vi "LDO Line Transient - Flat.vi"(11 "error in (no error)":errorcluster) -> (15 "error out":errorcluster)   [LabVIEW 2020]
uses:
  <instrlib>/niScope/Controls/niScope vertical coupling.ctl
  <instrlib>/niScope/Controls/niScope trigger source digital.ctl
  <instrlib>/niDCPower/nidcpower.llb/niDCPower Aperture Time Units.ctl
  <instrlib>/niDCPower/nidcpower.llb/niDCPower Source Mode.ctl
  <instrlib>/niDCPower/nidcpower.llb/niDCPower Output Function.ctl
  <instrlib>/niDCPower/nidcpower.llb/niDCPower Export Signal - Signal.ctl
  <instrlib>/niDCPower/nidcpower.llb/niDCPower Wait For Event - Event.ctl
  <instrlib>/niScope/Controls/niScope trigger slope.ctl
  <instrlib>/niScope/Configure/Trigger/niScope Configure Trigger Digital.vi
  <instrlib>/niScope/Acquire/Fetch/niScope Multi Fetch Cluster.vi
  <instrlib>/niScope/Utility/niScope Get Channel Name From String.vi
  <vilib>/gmath/NI_Gmath.lvlib
  LDO Line Transient.lvlib
  <vilib>/gmath/NumericalOptimization/Nonlinear Curve Fit LM formula string.vi
panel:
  out "Horizontal:Number of Records":i32=400000
  out "Horizontal:Min Sample Rate":dbl=1000000.0
  out "Measurement:Measure Record Length":i32=10
  out "Measurement:Aperture Time":dbl=4.9999999999999996e-06
  out "Source:Advanced:Source Delay":dbl=3.086419753086419e-08
  in  "Tab Control":T1(tab)=enum."Waveform"
  in  "Scope":refnum<k15>="PXI1Slot5"
  in  "Load SMU":refnum<k15>="SMU1"
  in  "Source SMU":refnum<k15>="SMU1"
  in  "Load SMU Voltage Limit (V)":dbl=8.0
  in  "Load SMU Voltage Limit Range (V)":dbl=8.0
  in  "Load SMU Current Level Range (A)":dbl=3.0
  in  "Load SMU Channel":string="1"
  in  "Load Current (A)":dbl=-0.05
  in  "Min. Record Length":i32=400000
  in  "Min. Sampling Rate":dbl=1000000.0
  in  "Trigger Modifier":i32(ring) items=["None", "Auto"]
  in  "Reference Position":dbl
  in  "Input Impedance":u32(ring) items=["1 Mega Ohm"=0, "50 Ohm"=2]
  in  "Trigger Delay (sec)":dbl
  in  "Max. Input Frequency (Hz)":dbl
  in  "Vertical Offset (V)":dbl
  in  "Probe Attentuation":dbl=1.0
  in  "Vertical Range (V)":dbl=5.0
  in  "Scope Channel":string="0"
  in  "Source SMU Current Limit (A)":dbl=0.2
  in  "Source SMU Transient Response":i32(ring)=1039 items=["Slow"=1041, "Normal"=1038, "Fast"=1039, "Custom"=1042]
  in  "Source SMU Record Length":i32=10
  in  "Source SMU Aperture Time (sec)":dbl=5e-06
  in  "Source SMU Current Limit Range (A)":dbl=0.2
  in  "Source SMU Voltage Level Range (V)":dbl=8.0
  in  "Source SMU Channel":string="0"
  in  "Source  SMU Steady State Voltage (V)":dbl=4.0
  in  "Vertical Coupling":T2 items=["AC", "DC", "Ground"]
  in  "Trigger Source":T3="VAL_PFI_0" caption="trigger source (RTSI 0)"
  in  "Recovery Level (V)":dbl=0.1
  in  "Vin2 Voltage Level Width (sec)":dbl=0.1
  in  "Source Voltage 2 - Vin2":dbl=5.0
  in  "Source Voltage 1 - Vin1":dbl=4.0
  out "Settling time (ms)":dbl=0.008841
  out "Mixed Signal Graph":cluster{waveform(dbl), waveform(dbl)}(graph)={{"t0"=timestamp(0 s since 1904-01-01), "dt"=4.9999999999999996e-06, "Y"=array[40000 elements]}, {"t0"=timestamp(0 s since 1904-01-01), "dt"=4.9999999999999996e-06, "Y"=array[40000 elements]}}
  out "Waveform Graph":dbl[](graph)
  out "Waveform(s)":T4(graph)={"relativeInitialX"=1e-06, "xIncrement"=1e-06, "wfm"=array[400000 elements]} caption="Instantaneous Load Transient Waveform"
  out "XY Graph 2":cluster{dbl[], dbl[]}[](graph)
  out "XY Graph":cluster{dbl[], "wfm":dbl[]}[](graph)
  # "Line Transient Measurement - Flat VI"
  # "Source SMU Config"
  # "Scope Config"
  # "Load SMU Config"
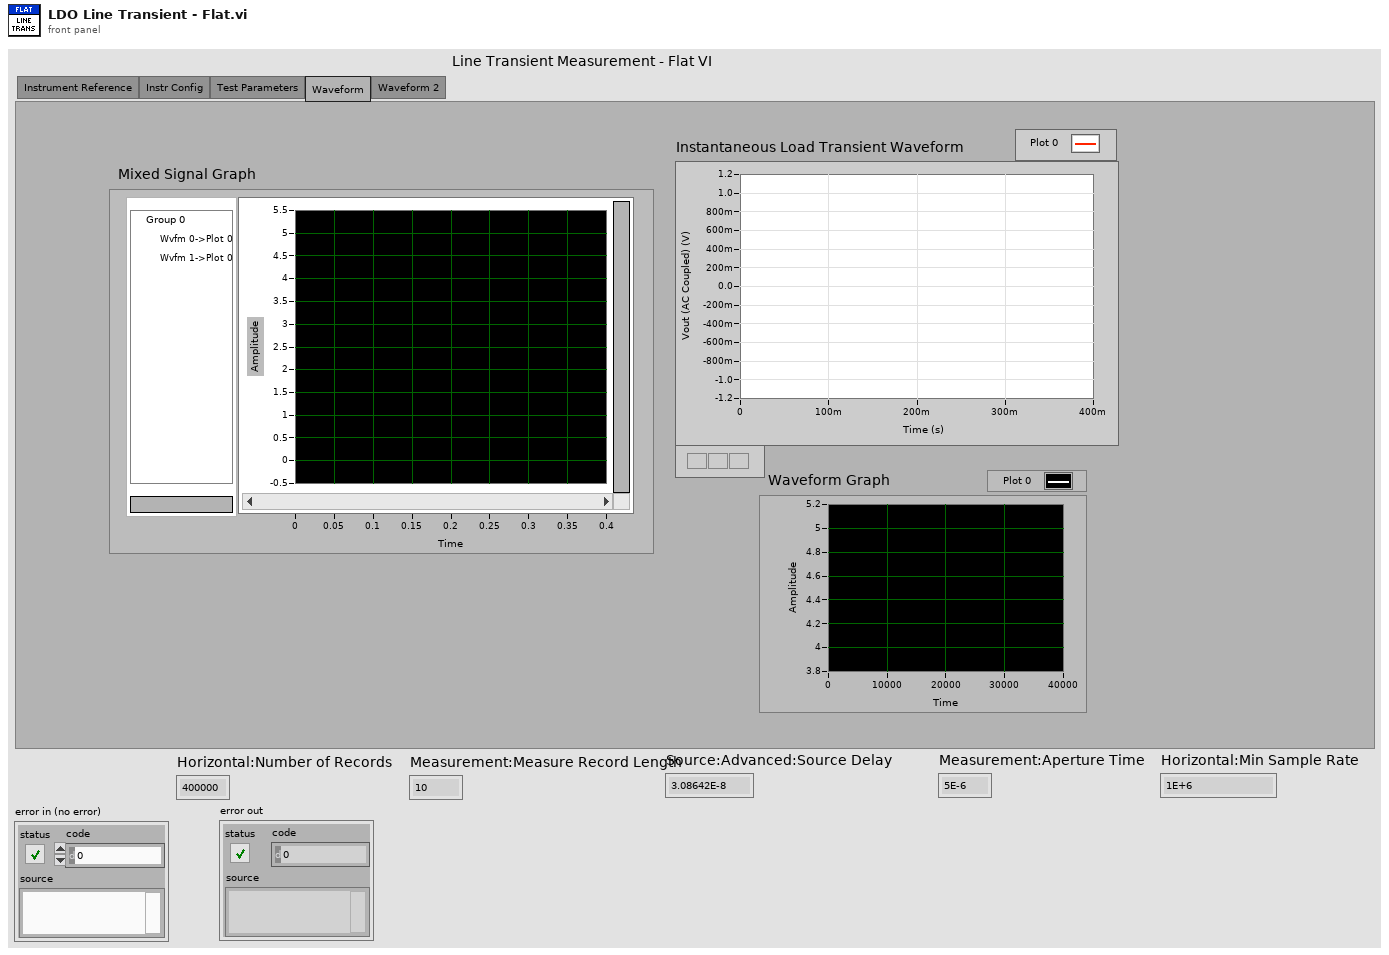
[diagram p1: front panel]
types:
  T1 = enum32{"Instrument Reference", "Instr Config", "Test Parameters", "Waveform", "Waveform 2"}
  T2 = typedef "niScope vertical coupling.ctl" = i32
  T3 = typedef "niScope trigger source digital.ctl" = string
  T4 = cluster{"relativeInitialX":dbl, "xIncrement":dbl, "wfm":dbl[]}
  T5 = typedef "niDCPower Output Function.ctl" = i32
  T6 = typedef "niDCPower Source Mode.ctl" = i32
  T7 = typedef "niScope trigger slope.ctl" = i32
  T8 = typedef "niDCPower Wait For Event - Event.ctl" = i32
  T9 = typedef "niDCPower Export Signal - Signal.ctl" = i32
  T10 = typedef "niDCPower Aperture Time Units.ctl" = i32
  T11 = cluster{"relativeInitialX":dbl, "xIncrement":dbl, "wfm":dbl[]}[]
  T12 = cluster{"model":string, "Parameters":string[], "x":string}
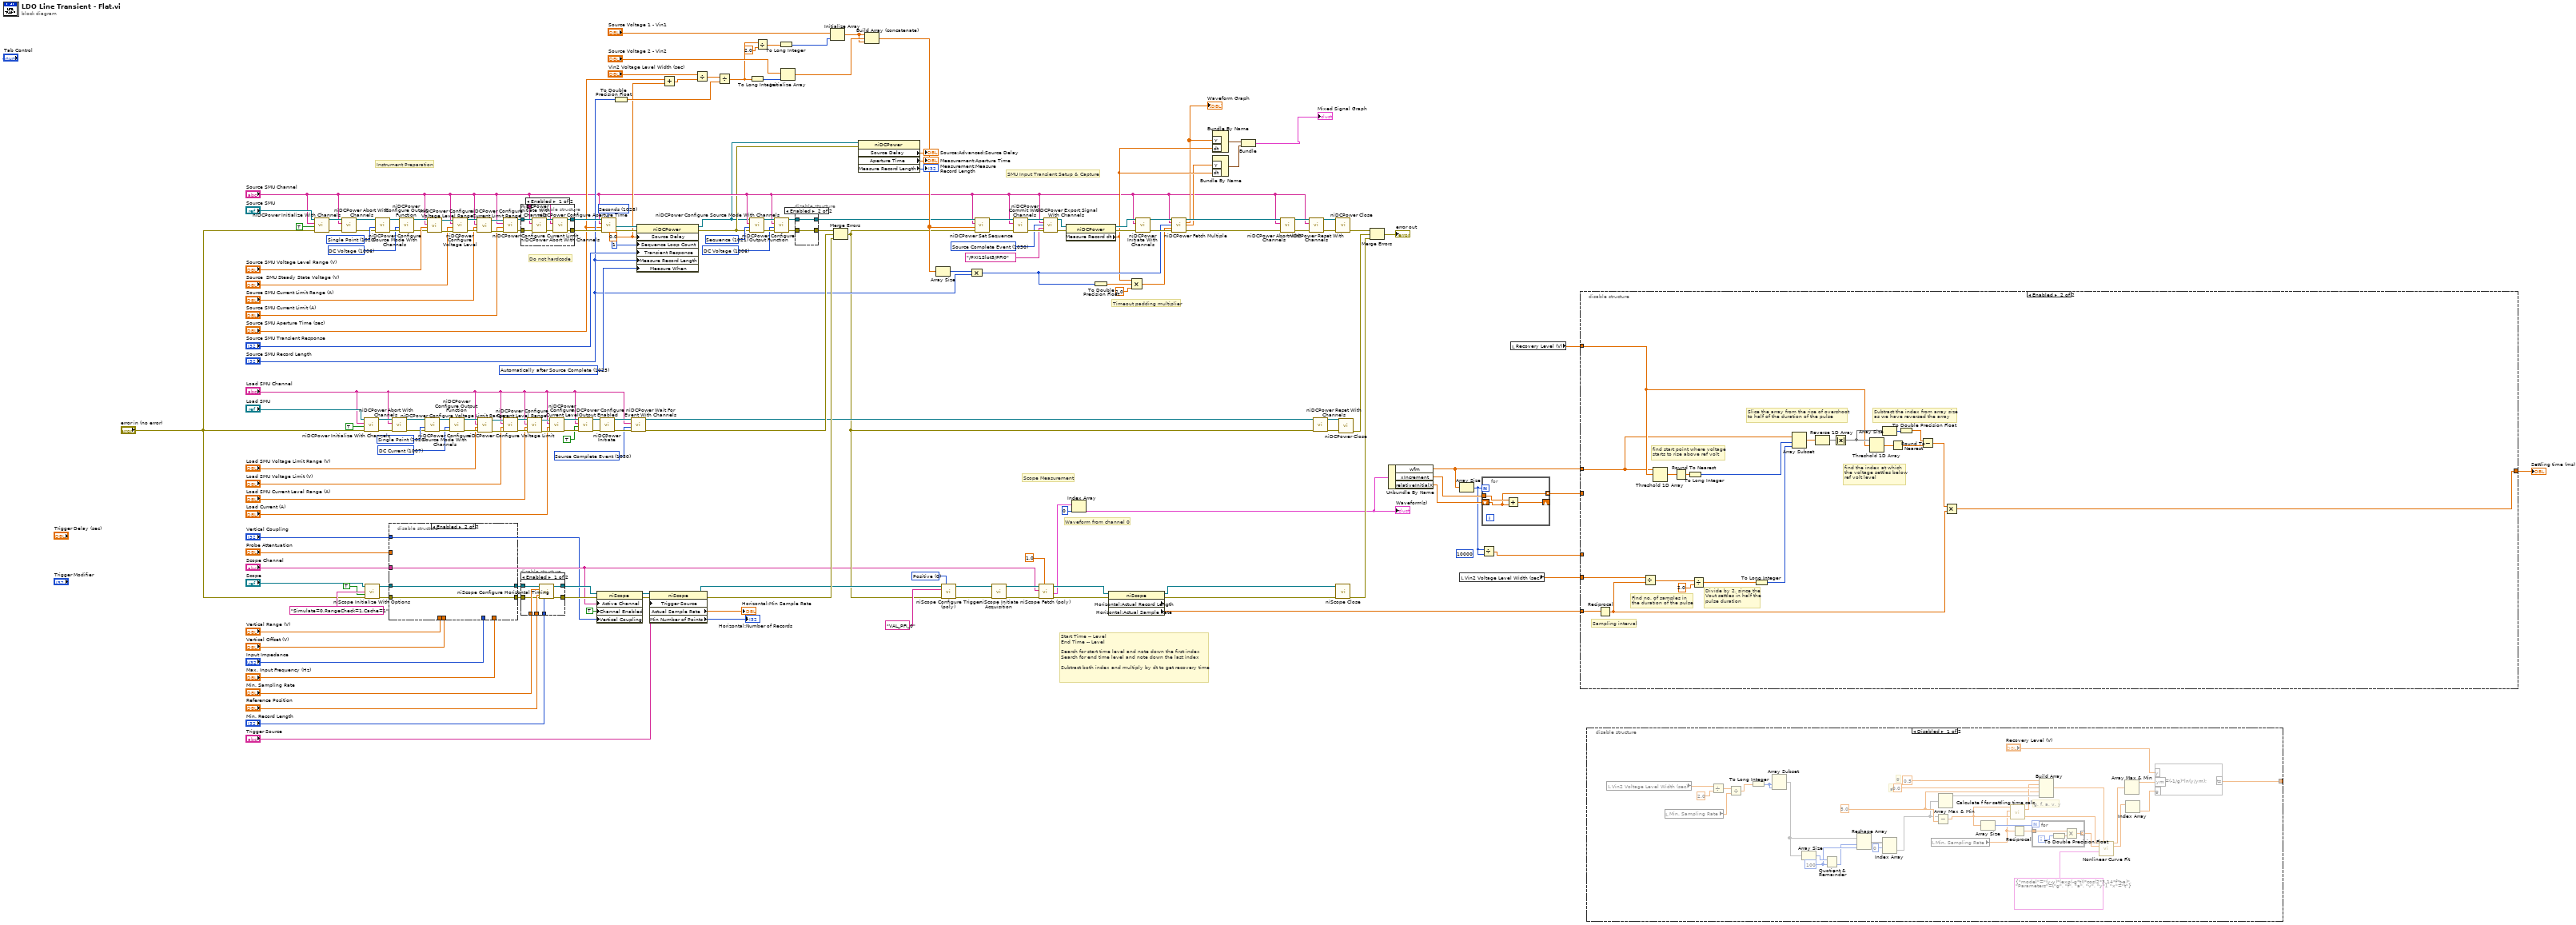
[diagram p0: block diagram]
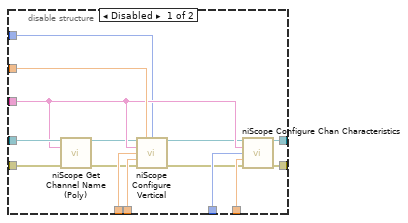
[diagram p2: hidden frame]
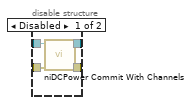
[diagram p4: hidden frame]
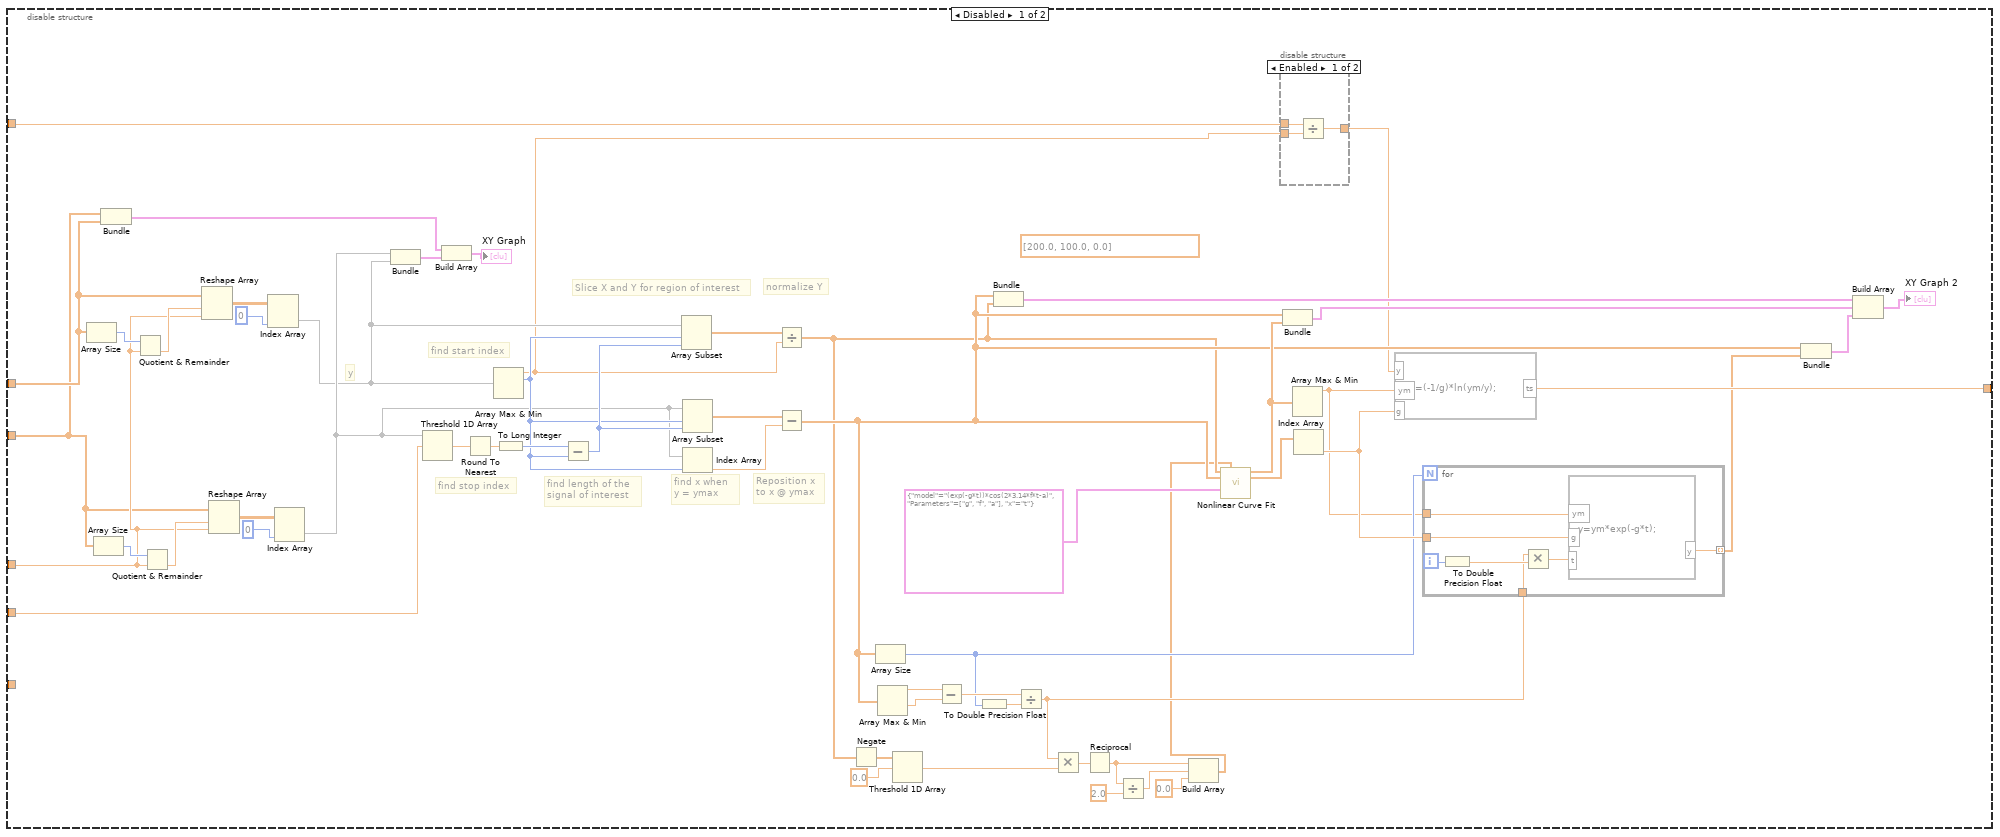
[diagram p5: hidden frame]
diagram:
  (unwired) 10000 ("y")
  w49 = T5 1006 items=["DC Voltage"=1006, "DC Current"=1007, "Pulse Voltage"=1049, "Pulse Current"=1050] ("output function")
  w50 = T6 1021 items=["Single Point"=1020, "Sequence"=1021] ("source mode")
  w43 = T7 0 items=["Positive", "Negative"] ("trigger slope")
  w76 = T8 1030 items=["Source Complete Event"=1030, "Measure Complete Event"=1031, "Sequence Iteration Complete Event"=1032, "Sequence Engine Done Event"=1033, "Pulse Complete Event"=1051, "Ready For Pulse Trigger Event"=1052] ("event")
  w110 = T9 1030 items=["Source Complete Event"=1030, "Measure Complete Event"=1031, "Sequence Iteration Complete Event"=1032, "Sequence Engine Done Event"=1033, "Pulse Complete Event"=1051, "Ready For Pulse Trigger Event"=1052, "Start Trigger"=1034, "Source Trigger"=1035, "Measure Trigger"=1036, "Sequence Advance Trigger"=1037, "Pulse Trigger"=1053] ("signal")
  w150 = T5 1007 items=["DC Voltage"=1006, "DC Current"=1007, "Pulse Voltage"=1049, "Pulse Current"=1050] ("output function")
  w151 = T6 1020 items=["Single Point"=1020, "Sequence"=1021] ("source mode")
  w159 = 1025 items=["Automatically after Source Complete"=1025, "On Demand"=1026, "On Measure Trigger"=1027] ("Measurement:Advanced:Measure When")
  w34 = 0.0 ("Source:Advanced:Source Delay")
  w166 = T10 1028 items=["Seconds"=1028, "Powerline Cycles"=1029] ("aperture time units")
  w169 = T5 1006 items=["DC Voltage"=1006, "DC Current"=1007, "Pulse Voltage"=1049, "Pulse Current"=1050] ("output function")
  w170 = T6 1020 items=["Single Point"=1020, "Sequence"=1021] ("source mode")
  # "Do not hardcode"
  # "Start Time -- Level\nEnd Time -- Level\n\nSearch for start time level and note down the first index\nSearch for end time level and note down the last index\n\nSubtract both index and multiply by dt to get recovery time"
  # "SMU Input Transient Setup & Capture"
  # "Scope Measurement"
  # "Waveform from channel 0"
  # "Timeout padding multiplier"
  # "Instrument Preparation"
  n1 = call <instrlib>:"niDCPower Initialize With Channels.vi"("error in (no error)"="error in (no error)", "reset (false)"=TRUE, "channels"="Source SMU Channel", "resource name"="Source SMU") -> ("error out"=w165:errorcluster, "instrument handle out"=w163:refnum<k15>)  [unwired: 1 in, 5 out]
  n2 = call <instrlib>:"niDCPower Abort With Channels.vi"("error in (no error)"=w165, "channel name"="Source SMU Channel", "instrument handle"=w163) -> ("error out"=w164:errorcluster, "instrument handle out"=w162:refnum<k15>)  [unwired: 7 in]
  n3 = call <instrlib>:"niDCPower Initialize With Channels.vi"("error in (no error)"="error in (no error)", "reset (false)"=TRUE, "channels"="Load SMU Channel", "resource name"="Load SMU") -> ("error out"=w147:errorcluster, "instrument handle out"=w145:refnum<k15>)  [unwired: 1 in, 5 out]
  n4 = call <instrlib>:"niScope Initialize With Options.vi"("resource name"="Scope", "option string"="Simulate=0,RangeCheck=1,Cache=1", "reset device"=TRUE, "error in"="error in (no error)") -> ("instrument handle"=w136:refnum<k15>, "error out"=w135:errorcluster)  [unwired: 10 in]
  n5 = call <instrlib>:"niDCPower Configure Source Mode With Channels.vi"("error in (no error)"=w164, "source mode"=w170, "instrument handle"=w162) -> ("error out"=w171:errorcluster, "instrument handle out"=w172:refnum<k15>)  [unwired: 7 in]
  n6 = disable-structure shown="Enabled" {
    disable-tunnel: w136 -> [w199 w200]
    disable-tunnel: w135 -> [w198 w201]
    disable-tunnel: "Probe Attentuation" -> [w197 _]
    disable-tunnel: "Vertical Range (V)" -> [w196 _]
    disable-tunnel: "Vertical Offset (V)" -> [w195 _]
    disable-tunnel: "Max. Input Frequency (Hz)" -> [w194 _]
    disable-tunnel: "Input Impedance" -> [w193 _]
    disable-tunnel: "Scope Channel" -> [w192 _]
    disable-tunnel: "Vertical Coupling" -> [w191 _]
    disable-tunnel: [w186 w201] -> w2
    disable-tunnel: [w185 w200] -> w1
    frame Disabled {
      n7 = call-poly <instrlib>:"niScope Get Channel Name (Poly).vi"("instrument handle"=w199, "index"=w192, "error in"=w198) -> ("instrument handle out"=w190:refnum<k15>, "error out"=w189:errorcluster)  [unwired: 10 in, 1 out]
      n8 = call <instrlib>:"niScope Configure Vertical.vi"("instrument handle"=w190, "probe attenuation"=w197, "vertical coupling"=w191, "channels"=w192, "vertical range"=w196, "vertical offset"=w195, "error in"=w189) -> ("instrument handle out"=w188:refnum<k15>, "error out"=w187:errorcluster)  [unwired: 7 in]
      n9 = call <instrlib>:"niScope Configure Chan Characteristics.vi"("instrument handle"=w188, "channels"=w192, "input impedance"=w193, "maximum input frequency"=w194, "error in"=w187) -> ("instrument handle out"=w185:refnum<k15>, "error out"=w186:errorcluster)  [unwired: 9 in]
    }
    frame Enabled {
    }
  }
  n10 = call <instrlib>:"niDCPower Abort With Channels.vi"("error in (no error)"=w147, "channel name"="Load SMU Channel", "instrument handle"=w145) -> ("error out"=w146:errorcluster, "instrument handle out"=w144:refnum<k15>)  [unwired: 7 in]
  n11 = call <instrlib>:"niDCPower Configure Output Function.vi"("error in (no error)"=w171, "output function"=w169, "instrument handle"=w172) -> ("error out"=w167:errorcluster, "instrument handle out"=w168:refnum<k15>)  [unwired: 7 in]
  n12 = call <instrlib>:"niDCPower Configure Source Mode With Channels.vi"("error in (no error)"=w146, "source mode"=w151, "instrument handle"=w144) -> ("error out"=w152:errorcluster, "instrument handle out"=w153:refnum<k15>)  [unwired: 7 in]
  n13 = call <instrlib>:"niDCPower Configure Voltage Level Range.vi"("error in (no error)"=w167, "voltage level range"="Source SMU Voltage Level Range (V)", "channel name"="Source SMU Channel", "instrument handle"=w168) -> ("error out"=w184:errorcluster, "instrument handle out"=w183:refnum<k15>)  [unwired: 6 in]
  n14 = call <instrlib>:"niDCPower Configure Output Function.vi"("error in (no error)"=w152, "output function"=w150, "instrument handle"=w153) -> ("error out"=w148:errorcluster, "instrument handle out"=w149:refnum<k15>)  [unwired: 7 in]
  n15 = call <instrlib>:"niDCPower Configure Voltage Level.vi"("error in (no error)"=w184, "voltage level"="Source  SMU Steady State Voltage (V)", "channel name"="Source SMU Channel", "instrument handle"=w183) -> ("error out"=w182:errorcluster, "instrument handle out"=w181:refnum<k15>)  [unwired: 6 in]
  n16 = call <instrlib>:"niDCPower Configure Current Limit Range.vi"("error in (no error)"=w182, "current limit range"="Source SMU Current Limit Range (A)", "channel name"="Source SMU Channel", "instrument handle"=w181) -> ("error out"=w180:errorcluster, "instrument handle out"=w179:refnum<k15>)  [unwired: 6 in]
  n17 = call <instrlib>:"niDCPower Configure Voltage Limit Range.vi"("error in (no error)"=w148, "voltage limit range"="Load SMU Voltage Limit Range (V)", "channel name"="Load SMU Channel", "instrument handle"=w149) -> ("error out"=w158:errorcluster, "instrument handle out"=w157:refnum<k15>)  [unwired: 6 in]
  n18 = call <instrlib>:"niDCPower Configure Current Limit.vi"("error in (no error)"=w180, "current limit"="Source SMU Current Limit (A)", "channel name"="Source SMU Channel", "instrument handle"=w179) -> ("error out"=w47:errorcluster, "instrument handle out"=w45:refnum<k15>)  [unwired: 6 in]
  n19 = call <instrlib>:"niDCPower Configure Voltage Limit.vi"("error in (no error)"=w158, "voltage limit"="Load SMU Voltage Limit (V)", "channel name"="Load SMU Channel", "instrument handle"=w157) -> ("error out"=w156:errorcluster, "instrument handle out"=w155:refnum<k15>)  [unwired: 6 in]
  n20 = disable-structure shown="Enabled" {
    disable-tunnel: w47 -> [w206 w209]
    disable-tunnel: [w205 w209] -> w46
    disable-tunnel: w45 -> [w204 w210]
    disable-tunnel: [w203 w210] -> w44
    disable-tunnel: "Source SMU Channel" -> [w202 _]
    frame Enabled {
      n21 = call <instrlib>:"niDCPower Initiate With Channels.vi"("error in (no error)"=w206, "channel name"=w202, "instrument handle"=w204) -> ("error out"=w208:errorcluster, "instrument handle out"=w207:refnum<k15>)  [unwired: 7 in]
      n22 = call <instrlib>:"niDCPower Abort With Channels.vi"("error in (no error)"=w208, "channel name"=w202, "instrument handle"=w207) -> ("error out"=w205:errorcluster, "instrument handle out"=w203:refnum<k15>)  [unwired: 7 in]
    }
    frame Disabled {
    }
  }
  n23 = disable-structure shown="Enabled" {
    disable-tunnel: "Min. Record Length" -> [w217 _]
    disable-tunnel: "Reference Position" -> [w216 _]
    disable-tunnel: "Min. Sampling Rate" -> [w215 _]
    disable-tunnel: [w214 w218] -> w11
    disable-tunnel: [w213 w219] -> w9
    disable-tunnel: w2 -> [w212 w218]
    disable-tunnel: w1 -> [w211 w219]
    frame Enabled {
      n24 = call <instrlib>:"niScope Configure Horizontal Timing.vi"("instrument handle"=w211, "min sample rate"=w215, "reference position"=w216, "error in"=w212, "min record length"=w217) -> ("instrument handle out"=w213:refnum<k15>, "error out"=w214:errorcluster)  [unwired: 9 in]
    }
    frame Disabled {
    }
  }
  n25 = call <instrlib>:"niDCPower Configure Current Level Range.vi"("error in (no error)"=w156, "current level range"="Load SMU Current Level Range (A)", "channel name"="Load SMU Channel", "instrument handle"=w155) -> ("error out"=w141:errorcluster, "instrument handle out"=w142:refnum<k15>)  [unwired: 6 in]
  n26 = call <instrlib>:"niDCPower Configure Current Level.vi"("error in (no error)"=w141, "current level"="Load Current (A)", "channel name"="Load SMU Channel", "instrument handle"=w142) -> ("error out"=w81:errorcluster, "instrument handle out"=w78:refnum<k15>)  [unwired: 6 in]
  n27 = call <instrlib>:"niDCPower Configure Output Enabled.vi"("error in (no error)"=w81, "output enabled"=TRUE, "channel name"="Load SMU Channel", "instrument handle"=w78) -> ("error out"=w80:errorcluster, "instrument handle out"=w83:refnum<k15>)  [unwired: 6 in]
  n28 = property class="niScope"(reference=w9, error in=w11, "Active Channel"="Scope Channel", "Channel Enabled"=TRUE ("Vertical:Channel Enabled"), "Vertical Coupling"="Vertical Coupling") -> (reference out=w8:refnum<k15>, error out=w10:errorcluster)
  n29 = call <instrlib>:"niDCPower Initiate.vi"("error in (no error)"=w80, "instrument handle"=w83) -> ("error out"=w79:errorcluster, "instrument handle out"=w82:refnum<k15>)  [unwired: 8 in]
  n30 = call <instrlib>:"niDCPower Configure Aperture Time.vi"("aperture time units"=w166, "error in (no error)"=w46, "aperture time"="Source SMU Aperture Time (sec)", "channel name"="Source SMU Channel", "instrument handle"=w44) -> ("error out"=w84:errorcluster, "instrument handle out"=w41:refnum<k15>)  [unwired: 5 out]
  n31 = To Double Precision Float(number="Source SMU Record Length") -> (double precision float=w38:dbl)
  n32 = call <instrlib>:"niDCPower Wait For Event With Channels.vi"("error in (no error)"=w79, "event"=w76, "channel name"="Load SMU Channel", "instrument handle"=w82) -> ("error out"=w74:errorcluster, "instrument handle out"=w57:refnum<k15>)  [unwired: 6 in]
  n33 = property class="niDCPower"(reference=w41, error in=w84, "Source Delay"=w34, "Sequence Loop Count"=1 ("Source:Advanced:Sequence Loop Count"), "Transient Response"="Source SMU Transient Response", "Measure Record Length"="Source SMU Record Length", "Measure When"=w159) -> (reference out=w12:refnum<k15>, error out=w13:errorcluster)
  n34 = property class="niScope"(reference=w8, error in=w10, "Trigger Source"="Trigger Source") -> (reference out=w71:refnum<k15>, error out=w73:errorcluster, "Actual Sample Rate"=→"Horizontal:Min Sample Rate":dbl, "Min Number of Points"=→"Horizontal:Number of Records":i32)
  n35 = Add(x="Source SMU Aperture Time (sec)", y=w34) -> (x+y=w35:dbl)
  n36 = Divide(x="Vin2 Voltage Level Width (sec)", y=w35) -> (x/y=w40:dbl)
  n37 = Divide(x=w40, y=w38) -> (x/y=w37:dbl)
  n38 = call <instrlib>:"niDCPower Configure Source Mode With Channels.vi"("error in (no error)"=w13, "source mode"=w50, "channel name"="Source SMU Channel", "instrument handle"=w12) -> ("error out"=w51:errorcluster, "instrument handle out"=w48:refnum<k15>)  [unwired: 6 in]
  n39 = To Long Integer(number=w37) -> (32bit integer=w122:i32)
  n40 = Divide(x=w37, y=2.0) -> (x/y=w118:dbl)
  n41 = call <instrlib>:"niDCPower Configure Output Function.vi"("error in (no error)"=w51, "output function"=w49, "channel name"="Source SMU Channel", "instrument handle"=w48) -> ("error out"=w18:errorcluster, "instrument handle out"=w16:refnum<k15>)  [unwired: 6 in]
  n42 = To Long Integer(number=w118) -> (32bit integer=w117:i32)
  n43 = Initialize Array("Source Voltage 2 - Vin2", w122) -> (w116:dbl[])
  n44 = disable-structure shown="Enabled" {
    disable-tunnel: w18 -> [w223 w224]
    disable-tunnel: [w222 w224] -> w17
    disable-tunnel: w16 -> [w221 w225]
    disable-tunnel: [w220 w225] -> w15
    frame Disabled {
      n45 = call <instrlib>:"niDCPower Commit With Channels.vi"("error in (no error)"=w223, "instrument handle"=w221) -> ("error out"=w222:errorcluster, "instrument handle out"=w220:refnum<k15>)  [unwired: 8 in]
    }
    frame Enabled {
    }
  }
  n46 = Initialize Array("Source Voltage 1 - Vin1", w117) -> (w115:dbl[])
  n47 = Merge Errors(w17, w74, w73) -> (w22:errorcluster)
  n48 = property class="niDCPower"(reference=w12, error in=w13) -> ("Source Delay"=→"Source:Advanced:Source Delay":dbl, "Aperture Time"=→"Measurement:Aperture Time":dbl, "Measure Record Length"=→"Measurement:Measure Record Length":i32)  [unwired: 2 out]
  n49 = Build Array (concatenate)(w115, w116, w115) -> (w106:dbl[])
  n50 = Array Size(array=w106) -> (size(s)=w105:i32)
  n51 = call-poly <instrlib>:"niScope Configure Trigger (poly).vi"("instrument handle"=w71, "trigger slope"=w43, "trigger source"=T3 "VAL_PFI_0", "error in"=w22) -> ("instrument handle out"=w72:refnum<k15>, "error out"=w86:errorcluster)  [unwired: 10 in]
  n52 = Compound Arithmetic op=MULTIPLY(w105, "Source SMU Record Length") -> (w98:i32)
  n53 = call <instrlib>:"niDCPower Set Sequence.vi"("error in (no error)"=w22, "values"=w106, "channel name"="Source SMU Channel", "instrument handle"=w15) -> ("error out"=w114:errorcluster, "instrument handle out"=w113:refnum<k15>)  [unwired: 1 in, 5 out]
  n54 = call <instrlib>:"niScope Initiate Acquisition.vi"("instrument handle"=w72, "error in"=w86) -> ("instrument handle out"=w69:refnum<k15>, "error out"=w85:errorcluster)  [unwired: 12 in]
  n55 = call <instrlib>:"niDCPower Commit With Channels.vi"("error in (no error)"=w114, "channel name"="Source SMU Channel", "instrument handle"=w113) -> ("error out"=w112:errorcluster, "instrument handle out"=w111:refnum<k15>)  [unwired: 7 in]
  n56 = call-poly <instrlib>:"niScope Fetch (poly).vi"("timeout"=1.0, "error in"=w85, "channels"="Scope Channel", "instrument handle"=w69) -> ("error out"=w87:errorcluster, "waveform"=w66:T11, "instrument handle out"=w67:refnum<k15>)  [unwired: 4 in, 1 out]
  n57 = call <instrlib>:"niDCPower Export Signal With Channels.vi"("instrument handle"=w111, "channel name"="Source SMU Channel", "signal"=w110, "output terminal"=tag "/PXI1Slot5/PFI0", "error in (no error)"=w112) -> ("instrument handle out"=w107:refnum<k15>, "error out"=w108:errorcluster)  [unwired: 9 in]
  n58 = property class="niDCPower"(reference=w107, error in=w108) -> (reference out=w101:refnum<k15>, error out=w102:errorcluster, "Measure Record dt"=w90:dbl)
  n59 = Index Array(array=w66, index=0) -> (element=w33:T4)
  "Waveform(s)" <- w33
  n60 = To Double Precision Float(number=w98) -> (double precision float=w103:dbl)
  n61 = property class="niScope" props=["Horizontal:Actual Record Length", "Horizontal:Actual Sample Rate"](reference=w67, error in=w87) -> (reference out=w63:refnum<k15>, error out=w64:errorcluster, "Horizontal:Actual Sample Rate"=w23:dbl)  [unwired: 1 out]
  n62 = Compound Arithmetic op=MULTIPLY(w90, w103, 2.0 ("value")) -> (w97:dbl)
  n63 = call <instrlib>:"niDCPower Initiate With Channels.vi"("error in (no error)"=w102, "channel name"="Source SMU Channel", "instrument handle"=w101) -> ("error out"=w100:errorcluster, "instrument handle out"=w99:refnum<k15>)  [unwired: 7 in]
  n64 = call <instrlib>:"niDCPower Fetch Multiple.vi"("instrument handle"=w99, "channel name"="Source SMU Channel", "count (1)"=w98, "timeout (sec)"=w97, "error in (no error)"=w100) -> ("instrument handle out"=w95:refnum<k15>, "voltage measurements"=w54:dbl[], "current measurements"=w89:dbl[], "error out"=w96:errorcluster)  [unwired: 7 out]
  "Waveform Graph" <- w54
  n65 = Bundle By Name("Y"=w54, "dt"=w90) -> (w88:waveform(dbl))  [unwired: 1 out]
  n66 = Bundle By Name("Y"=w89, "dt"=w90) -> (w53:waveform(dbl))  [unwired: 1 out]
  n67 = Bundle(w88, w53) -> (→"Mixed Signal Graph":cluster{waveform(dbl), waveform(dbl)})  [unwired: 1 in]
  n68 = call <instrlib>:"niDCPower Abort With Channels.vi"("error in (no error)"=w96, "channel name"="Source SMU Channel", "instrument handle"=w95) -> ("error out"=w93:errorcluster, "instrument handle out"=w91:refnum<k15>)  [unwired: 7 in]
  n69 = call <instrlib>:"niDCPower Reset With Channels.vi"("error in (no error)"=w93, "channel name"="Source SMU Channel", "instrument handle"=w91) -> ("error out"=w92:errorcluster, "instrument handle out"=w94:refnum<k15>)  [unwired: 7 in]
  n70 = call <instrlib>:"niDCPower Reset With Channels.vi"("error in (no error)"=w22, "instrument handle"=w57) -> ("error out"=w58:errorcluster, "instrument handle out"=w59:refnum<k15>)  [unwired: 8 in]
  n71 = call <instrlib>:"niDCPower Close.vi"("error in (no error)"=w92, "instrument handle"=w94) -> ("error out"=w62:errorcluster)  [unwired: 9 out]
  n72 = call <instrlib>:"niScope Close.vi"("instrument handle"=w63, "error in"=w64) -> ("error out"=w61:errorcluster)  [unwired: 13 in]
  n73 = call <instrlib>:"niDCPower Close.vi"("error in (no error)"=w58, "instrument handle"=w59) -> ("error out"=w56:errorcluster)  [unwired: 9 out]
  n74 = Merge Errors(w62, w56, w61) -> (→"error out":errorcluster)
  n75 = Unbundle By Name(w33) -> ("wfm"=w28:dbl[], "xIncrement"=w31:dbl, "relativeInitialX"=w32:dbl)
  n76 = Array Size(array=w28) -> (size(s)=w26:i32)
  n77 = local read "Vin2 Voltage Level Width (sec)"() -> (w25:dbl)
  n78 = Divide(x=w26, y=w26) -> (x/y=w29:dbl)
  n79 = for {
    N: w26 -> [_]
    tunnel: w31 -> [w228]
    shift-right: [w227] -> _
    shift-left: w32 -> [w226]
    tunnel: [w226] -> w27 mode=indexing
    n80 = Add(x=w228, y=w226) -> (x+y=w227:dbl)
  }
  n81 = local read "Recovery Level (V)"() -> (w24:dbl)
  n82 = disable-structure shown="Enabled" {
    disable-tunnel: [w274 w300] -> w30
    disable-tunnel: w29 -> [w255 _]
    disable-tunnel: w28 -> [w238 w297]
    disable-tunnel: w27 -> [w237 _]
    disable-tunnel: w25 -> [w230 w296]
    disable-tunnel: w24 -> [w229 w298]
    disable-tunnel: w23 -> [_ w299]
    frame Disabled {
      (unwired) dbl[] [200.0, 100.0, 0.0] ("initial parameters")
      # "find x when \ny = ymax"
      # "Reposition x \nto x @ ymax"
      # "normalize Y"
      # "Slice X and Y for region of interest"
      # "find length of the \nsignal of interest"
      # "find stop index"
      # "find start index"
      # "y"
      n83 = Array Size(array=w238) -> (size(s)=w264:i32)
      n84 = Array Size(array=w237) -> (size(s)=w268:i32)
      n85 = Bundle(w237, "wfm"=w238) -> (w235:cluster{dbl[], "wfm":dbl[]})  [unwired: 1 in]
      n86 = Quotient & Remainder(x=w264, y=w255) -> (floor(x/y)=w263:dbl)  [unwired: 1 out]
      n87 = Quotient & Remainder(x=w268, y=w255) -> (floor(x/y)=w267:dbl)  [unwired: 1 out]
      n88 = Reshape Array(w238, w263, w255) -> (w262:dbl[][])
      n89 = Reshape Array(w237, w267, w255) -> (w266:dbl[][])
      n90 = Index Array(array=w262, index (col)=0 ("index (row)")) -> (element=w261:dbl[])  [unwired: 1 in]
      n91 = Index Array(array=w266, index (col)=0 ("index (row)")) -> (element=w265:dbl[])  [unwired: 1 in]
      n92 = Bundle(w265, "wfm"=w261) -> (w272:cluster{dbl[], "wfm":dbl[]})  [unwired: 1 in]
      n93 = Threshold 1D Array(2:w230, 3:w265) -> (0:w283:dbl)  [unwired: 1 in]
      n94 = Build Array(w235, w272) -> (→"XY Graph":cluster{dbl[], "wfm":dbl[]}[])
      n95 = Round To Nearest(number=w283) -> (nearest integer value=w284:dbl)
      n96 = Array Max & Min(array=w261) -> (max value=w233:dbl, max index (indices)=w278:i32)  [unwired: 2 out]
      n97 = To Long Integer(number=w284) -> (32bit integer=w282:i32)
      n98 = Subtract(x=w282, y=w278) -> (x-y=w281:i32)
      n99 = Array Subset(array=w261, index=w278, length=w281) -> (w280:dbl[])
      n100 = Array Subset(array=w265, index=w278, length=w281) -> (w279:dbl[])
      n101 = Index Array(array=w265, index=w278) -> (element=w277:dbl)
      n102 = Divide(x=w280, y=w233) -> (x/y=w248:dbl[])
      n103 = Subtract(x=w279, y=w277) -> (x-y=w254:dbl[])
      n104 = Negate(x=w248) -> (-x=w247:dbl[])
      n105 = Array Size(array=w254) -> (size(s)=w250:i32)
      n106 = Array Max & Min(array=w254) -> (max value=w253:dbl, min value=w252:dbl)  [unwired: 2 out]
      n107 = Threshold 1D Array(2:0.0 ("threshold y"), 3:w247) -> (0:w245:dbl)  [unwired: 1 in]
      n108 = Subtract(x=w253, y=w252) -> (x-y=w251:dbl)
      n109 = To Double Precision Float(number=w250) -> (double precision float=w249:dbl)
      n110 = Bundle(w254, w248) -> (w273:cluster{dbl[], dbl[]})  [unwired: 1 in]
      n111 = Divide(x=w251, y=w249) -> (x/y=w244:dbl)
      n112 = Multiply(x=w244, y=w245) -> (x*y=w243:dbl)
      n113 = Reciprocal(x=w243) -> (1/x=w242:dbl)
      n114 = Divide(x=w242, y=2.0) -> (x/y=w240:dbl)
      n115 = Build Array(w242, w240, 0.0 ("element")) -> (w231:dbl[])
      n116 = call-poly <vilib>:"Nonlinear Curve Fit.vi"("Y"=w248, "initial parameters"=w231, "X"=w254, "model description"=T12 {"model"="(exp(-g*t))*cos(2*3.14*f*t-a)", "Parameters"=["g", "f", "a"], "x"="t"}) -> ("best nonlinear fit"=w271:dbl[], "best fit parameters"=w275:dbl[])  [unwired: 7 in, 3 out]
      n117 = disable-structure shown="Enabled" {
        disable-tunnel: w229 -> [w287 w288]
        disable-tunnel: [w286 w288] -> w234
        disable-tunnel: w233 -> [w285 _]
        frame Enabled {
          n118 = Divide(x=w287, y=w285) -> (x/y=w286:dbl)
        }
        frame Disabled {
        }
      }
      n119 = Bundle(w254, "best nonlinear fit"=w271) -> (w269:cluster{dbl[], "best nonlinear fit":dbl[]})  [unwired: 1 in]
      n120 = Array Max & Min(array=w271) -> (max value=w232:dbl)  [unwired: 3 out]
      n121 = Index Array(array=w275) -> (element=w258:dbl)  [unwired: 1 in]
      n122 = formula code="ts =(-1/g)*ln(ym/y);"("y"=w234, "ym"=w232, "g"=w258) -> ("ts"=w274:dbl)
      n123 = for {
        N: w250 -> [_]
        tunnel: [w294] -> w257 mode=indexing
        tunnel: w258 -> [w291]
        tunnel: w232 -> [w290]
        tunnel: w244 -> [w289]
        i -> [w295]
        n124 = To Double Precision Float(number=w295) -> (double precision float=w292:dbl)
        n125 = Multiply(x=w289, y=w292) -> (x*y=w293:dbl)
        n126 = formula code="y=ym*exp(-g*t);"("g"=w291, "ym"=w290, "t"=w293) -> ("y"=w294:dbl)
      }
      n127 = Bundle(w254, w257) -> (w256:cluster{dbl[], dbl[]})  [unwired: 1 in]
      n128 = Build Array(w273, w269, w256) -> (→"XY Graph 2":cluster{dbl[], "best nonlinear fit":dbl[]}[])
    }
    frame Enabled {
      # "Subtract the index from array size\nas we have reversed the array"
      # "Sampling interval"
      # "find the index at which \nthe voltage settles below\nref volt level"
      # "Slice the array from the rise of overshoot\nto half of the duration of the pulse"
      # "Divide by 2, since the\nVout settles in half the\npulse duration"
      # "Find no. of samples in \nthe duration of the pulse"
      # "find start point where voltage\nstarts to rise above ref volt"
      n129 = Reciprocal(x=w299) -> (1/x=w308:dbl)
      n130 = Divide(x=w296, y=w308) -> (x/y=w314:dbl)
      n131 = Threshold 1D Array(2:w298, 3:w297) -> (0:w316:dbl)  [unwired: 1 in]
      n132 = Round To Nearest(number=w316) -> (nearest integer value=w315:dbl)
      n133 = To Long Integer(number=w315) -> (32bit integer=w307:i32)
      n134 = Divide(x=w314, y=2.0) -> (x/y=w312:dbl)
      n135 = To Long Integer(number=w312) -> (32bit integer=w311:i32)
      n136 = Array Subset(array=w297, index=w307, length=w311) -> (w306:dbl[])
      n137 = Reverse 1D Array(array=w306) -> (reversed array=w310:dbl[])
      n138 = Absolute Value(x=w310) -> (abs(x)=w303:dbl[])
      n139 = Threshold 1D Array(2:w298, 3:w303) -> (0:w309:dbl)  [unwired: 1 in]
      n140 = Array Size(array=w303) -> (size(s)=w302:i32)
      n141 = Round To Nearest(number=w309) -> (nearest integer value=w305:dbl)
      n142 = To Double Precision Float(number=w302) -> (double precision float=w301:dbl)
      n143 = Subtract(x=w301, y=w305) -> (x-y=w304:dbl)
      n144 = Multiply(x=w304, y=w308) -> (x*y=w300:dbl)
    }
  }
  "Settling time (ms)" <- w30
  n145 = disable-structure shown="Disabled" {
    disable-tunnel: [w317 _] -> _
    frame Disabled {
      w323 = 100 ("y")
      w327 = 5.0 ("element")
      # "a"
      # "g"
      # "g, f, a, v, y"
      n146 = local read "Vin2 Voltage Level Width (sec)"() -> (w343:dbl)
      n147 = local read "Min. Sampling Rate"() -> (w325:dbl)
      n148 = Divide(x=w343, y=2.0) -> (x/y=w346:dbl)
      n149 = Divide(x=w346, y=w325) -> (x/y=w345:dbl)
      n150 = To Long Integer(number=w345) -> (32bit integer=w344:i32)
      n151 = Array Subset(index=w344, length=w344) -> (w319:void[])  [unwired: 1 in]
      n152 = Array Size(array=w319) -> (size(s)=w324:i32)
      n153 = Quotient & Remainder(x=w324, y=w323) -> (floor(x/y)=w322:i32)  [unwired: 1 out]
      n154 = Reshape Array(w319, w322, w323) -> (w321:void[][])
      n155 = Index Array(array=w321, index (row)=0) -> (element=w318:void[])  [unwired: 1 in]
      n156 = local read "Min. Sampling Rate"() -> (w328:dbl)
      n157 = Subtract(x=w318, y=w327) -> (x-y=w336:dbl)
      n158 = Array Max & Min(array=w318) -> (max value=w338)  [unwired: 3 out]
      n159 = Array Size(array=w336) -> (size(s)=w339:i32)
      n160 = call "Calculate f for settling time calc.vi"("Sampling Freq (Hz)"=w328, "Scope Waveform"=w336) -> ("Frequency 'f'"=w335:dbl)  [unwired: 3 in]
      n161 = Reciprocal(x=w328) -> (1/x=w341:dbl)
      n162 = for {
        N: w339 -> [_]
        tunnel: w341 -> [w351]
        tunnel: [w348] -> w340 mode=indexing
        i -> [w350]
        n163 = To Double Precision Float(number=w350) -> (double precision float=w349:dbl)
        n164 = Multiply(x=w351, y=w349) -> (x*y=w348:dbl)
      }
      n165 = Build Array(0.5 ("element"), w335, 0.0 ("element"), w327, w338) -> (w333:dbl[])
      n166 = call-poly <vilib>:"Nonlinear Curve Fit.vi"("Y"=w336, "initial parameters"=w333, "X"=w340, "model description"=T12 {"model"="(y-v)*(exp(-g*t))*cos(2*3.14*f*t-a)", "Parameters"=["g", "f", "a", "v", "y"], "x"="t"}) -> ("best nonlinear fit"=w332:dbl[], "best fit parameters"=w331:dbl[])  [unwired: 7 in, 3 out]
      n167 = Array Max & Min(array=w332) -> (max value=w330:dbl)  [unwired: 3 out]
      n168 = Index Array(array=w331) -> (element=w329:dbl)  [unwired: 1 in]
      n169 = formula code="ts =(-1/g)*ln(y/ym);"("y"="Recovery Level (V)", "ym"=w330, "g"=w329) -> ("ts"=w317:dbl)
    }
    frame Enabled {
    }
  }
